vi "RichToFlatgoogle_protobuf_Any.vi"(5 "OutputClusterType":T1, 11 "InputCluster":T2) -> (3 "OutputCluster":T1)   [LabVIEW 2020, in "Measurement Plugin Measurement Server Internal.lvlib"]
uses:
  Measurement Plugin Measurement Server Internal.lvlib
  google_protobuf_Any.ctl
  google_protobuf_Any_Flat.ctl
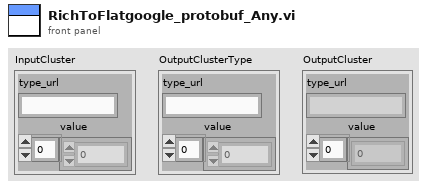
[diagram p1: front panel]
types:
  T1 = typedef "Measurement Plugin Measurement Server Internal.lvlib/google_protobuf_Any_Flat.ctl" = cluster{"type_url":string, "value":u8[]}
  T2 = typedef "Measurement Plugin Measurement Server Internal.lvlib/google_protobuf_Any.ctl" = cluster{"type_url":string, "value":u8[]}
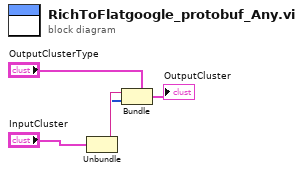
[diagram p0: block diagram]
diagram:
  n1 = Unbundle "Unbundle"("InputCluster") -> ("type_url"=w2:string, "value"=w1:u8[])
  n2 = Bundle "Bundle"(cluster="OutputClusterType", "type_url"=w2, "value"=w1) -> (→"OutputCluster":T1)
